vi "Remove.vi"(11 "TypedCircularBuffer in":refnum<class "LogCircularBuffer.lvclass">) -> (1 "invalid?":bool, 2 "element":T1, 3 "TypedCircularBuffer out":refnum<class "LogCircularBuffer.lvclass">)   [LabVIEW 2024, in "LogCircularBuffer.lvclass"]
uses:
  LogCircularBuffer.lvclass
  Type.ctl
  RQMHCore/ErrorReporting/Record/LogRecord.lvclass
  LogCircularBuffer.lvclass/LogCircularBuffer.ctl
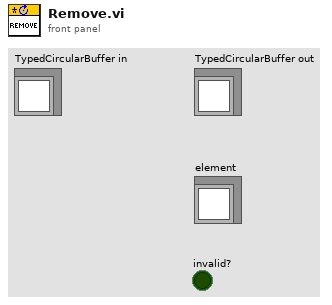
[diagram p1: front panel]
types:
  T1 = typedef "LogCircularBuffer.lvclass/Type.ctl" = refnum<class "LogRecord.lvclass">
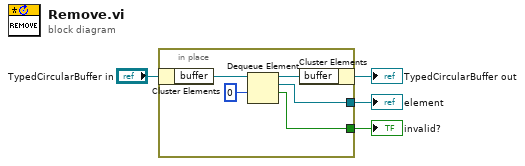
[diagram p0: block diagram]
diagram:
  n1 = in-place {
    in-place-border: [w8] -> w3
    in-place-border: [w7] -> w2
    n2 = in-place-cluster #1("TypedCircularBuffer in") -> ("buffer"=w9:refnum<queue>)
    n3 = Dequeue Element(queue=w9, timeout in ms (-1)=0) -> (queue out=w6:refnum<queue>, element=w8:T1, timed out?=w7:bool)  [unwired: 1 in, 1 out]
    n4 = in-place-cluster #1("buffer"=w6) -> (→"TypedCircularBuffer out":refnum<class "LogCircularBuffer.lvclass">)
  }
  "element" <- w3
  "invalid?" <- w2
